vi "DISP_WIND_TRAC_MEM_STAT.vi"(0 "VISA IN":refnum<visa-resource-name>, 1 "Trace":i32=1, 2 "ON | OFF":bool, 5 "error in":errorcluster, 7 "Window":i32=1) -> (14 "VISA Out":refnum<visa-resource-name>, 19 "error out":errorcluster)   [LabVIEW 2018, in "PNA-X.lvlib"]
doc: "DISPlay:WINDow<wnum>:TRACe<tnum>MEMory[:STATe] <ON | OFF> \n(Read-Write) Turns the memory trace ON or OFF. \nParameters \n<wnum> Any existing window number. If unspecified, value is set to 1. \n<tnum> Any existing trace number; if unspecified, value is set to 1 \n<ON | OFF> ON (or 1) - turns the memory trace ON. \nOFF (or 0) - turns the memory trace OFF. \nExamples DISP:WIND:TRAC:MEM ON \ndisplay:window2:trace2:memory:state off \nQuery Syntax DISPlay:WIND<wnum>:TRACe<tnum>:MEMory[:STATe]? \nReturn Type Boolean (1 = ON, 0 = OFF) \nDefault OFF"
uses:
  PNA-X.lvlib
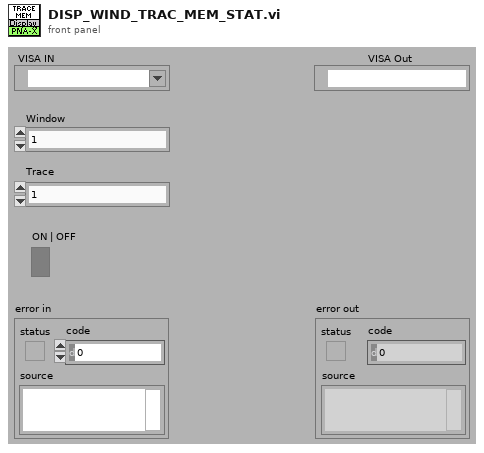
[diagram p1: front panel]
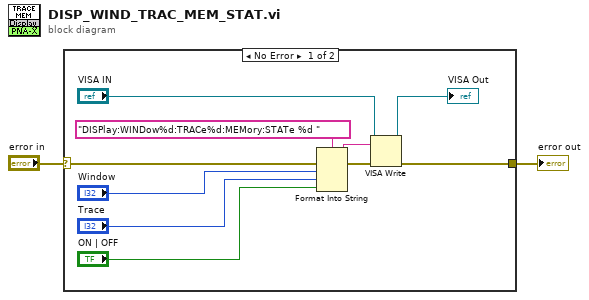
[diagram p0: block diagram]
diagram:
  n1 = case shown="No Error" "error in" {
    selector: "error in" -> [w12 w13]
    tunnel: [w7 w13] -> w1
    frame No Error {
      n2 = Format Into String(format string="DISPlay:WINDow%d:TRACe%d:MEMory:STATe %d " ("Cmdline"), error in=w12, "Window", "Trace", "ON | OFF") -> (resulting string=w10:string, error out=w11:errorcluster)  [unwired: 1 in]
      n3 = VISA Write(VISA resource name="VISA IN", write buffer=w10, error in (no error)=w11) -> (VISA resource name out=→"VISA Out":refnum<visa-resource-name>, error out=w7:errorcluster)  [unwired: 1 out]
    }
    frame Error {
    }
  }
  "error out" <- w1
